vi "Complex Compact Tri-Matrix Linear Eqs.vi"(2 "Known Vector":cdb[](array[numeric]) format="%.2f", 3 "Triangular Compact Array":cluster{"Compact Array":cdb[], "array type":i32} {"array type" items=["lower triangular", "upper triangular"]; "Compact Array" format="%.2f"}) -> (0 "error":i32, 1 "Solution Vector":cdb[](array[numeric]) format="%.2f")   [LabVIEW 2020, in "NI_AALBase.lvlib"]
doc: "Solves a linear system of simultaneous equations, if possible. The system is solved using the method known as L-U decomposition."
uses:
  NI_AALBase.lvlib
  <resource>/lvanlys.dll
panel:
  # "Complex Compact Tri-Matrix Linear Eqs"
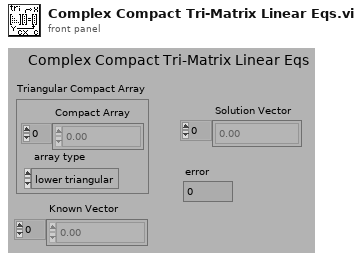
[diagram p1: front panel]
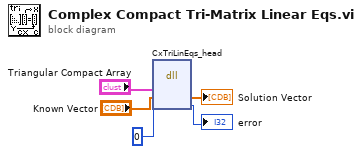
[diagram p0: block diagram]
diagram:
  n1 = dll-call lib="C:/Program Files (x86)/National Instruments/LabVIEW 2020/resource/lvanlys.*" fn="CxTriLinEqs_head"("Triangular Compact Array"="Triangular Compact Array", "Known Vector"="Known Vector", 0) -> ("Known Vector"=→"Solution Vector":cdb[], →"error":i32)  [unwired: 5 in, 2 out]
